vi "PinPointToRect.vi"(8 "错误输入":errorcluster, 10 "point":cluster{"x":i16, "y":i16} caption="点", 11 "rect":T2 caption="矩形") -> (0 "错误输出":errorcluster, 1 "edge":T1 caption="边缘", 2 "pinned point":cluster{"x":i16, "y":i16} caption="锁定点")   [LabVIEW 2012, in "Picture Box Tools.lvlib" / "Rect Tools.lvlib"]
uses:
  Rect Tools.lvlib
  EdgeEnum.ctl
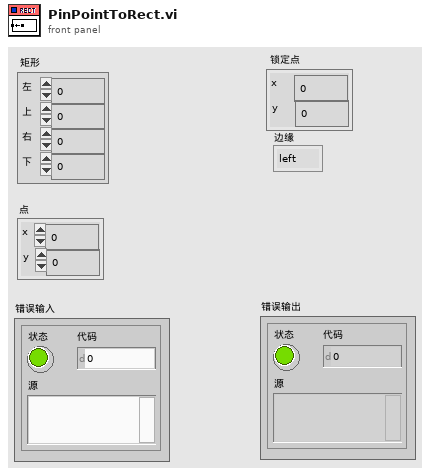
[diagram p1: front panel]
types:
  T1 = typedef "Picture Box Tools.lvlib/Rect Tools.lvlib/EdgeEnum.ctl" = enum16{"left", "top", "right", "bottom"}
  T2 = cluster{"left":i16, "top":i16, "right":i16, "bottom":i16}
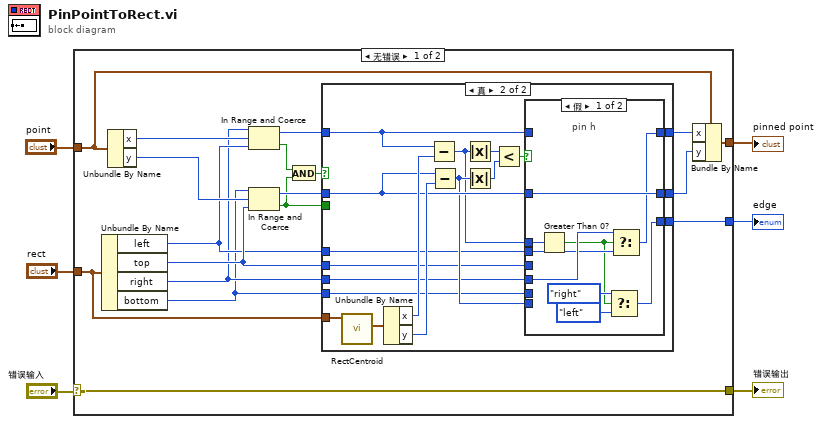
[diagram p0: block diagram]
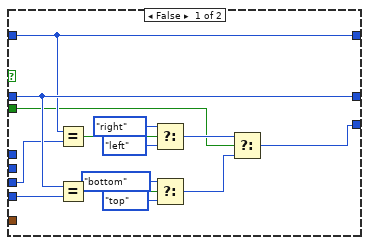
[diagram p2: hidden frame]
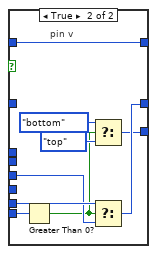
[diagram p3: hidden frame]
diagram:
  n1 = case shown="无错误" "错误输入" {
    selector: "错误输入" -> [w11 w75]
    tunnel: [w11 w75] -> w5
    tunnel: "point" -> [w10 _]
    tunnel: "rect" -> [w9 _]
    tunnel: [w8 _] -> w2
    tunnel: [w7 _] -> w1
    frame No Error {
      n2 = Unbundle By Name(w9) -> ("left"=w15:i16, "top"=w16:i16, "right"=w13:i16, "bottom"=w12:i16)
      n3 = Unbundle By Name(w10) -> ("x"=w24:i16, "y"=w23:i16)
      n4 = In Range and Coerce(upper limit=w13, x=w24, lower limit=w15) -> (coerced(x)=w20:i16, In Range?=w22:bool)
      n5 = In Range and Coerce(upper limit=w12, x=w23, lower limit=w16) -> (coerced(x)=w19:i16, In Range?=w14:bool)
      n6 = And(x=w22, y=w14) -> (x .and. y?=w21:bool)
      n7 = case shown="真" w21 {
        tunnel: w20 -> [w29 w48]
        tunnel: w19 -> [w34 w49]
        tunnel: [w29 w47] -> w18
        tunnel: [w34 w46] -> w17
        tunnel: w9 -> [_ w56]
        tunnel: w12 -> [w35 w40]
        tunnel: w16 -> [_ w42]
        tunnel: w13 -> [w30 w41]
        tunnel: w15 -> [_ w43]
        tunnel: [w26 w39] -> w7
        tunnel: w14 -> [w25 _]
        frame False {
          n8 = Equal?(x=w29, y=w30) -> (x = y?=w33:bool)
          n9 = Equal?(x=w34, y=w35) -> (x = y?=w36:bool)
          n10 = Select(t=EdgeEnum."right" ("edge"), s=w33, f=EdgeEnum."left" ("edge")) -> (s? t:f=w28:T1)
          n11 = Select(t=EdgeEnum."bottom" ("edge"), s=w36, f=EdgeEnum."top" ("edge")) -> (s? t:f=w27:T1)
          n12 = Select(t=w28, s=w25, f=w27) -> (s? t:f=w26:T1)
        }
        frame True {
          n13 = call "RectCentroid.vi"("Rect In"=w56) -> ("point"=w55:cluster{"x":i16, "y":i16})  [unwired: 8 in, 2 out]
          n14 = Unbundle By Name(w55) -> ("x"=w54:i16, "y"=w53:i16)
          n15 = Subtract(x=w48, y=w54) -> (x-y=w44:i16)
          n16 = Subtract(x=w49, y=w53) -> (x-y=w45:i16)
          n17 = Absolute Value(x=w44) -> (abs(x)=w51:i16)
          n18 = Absolute Value(x=w45) -> (abs(x)=w52:i16)
          n19 = Less?(x=w51, y=w52) -> (x < y?=w50:bool)
          n20 = case shown="假" w50 {
            tunnel: w49 -> [w65 _]
            tunnel: w48 -> [_ w74]
            tunnel: [w64 w74] -> w47
            tunnel: [w65 w73] -> w46
            tunnel: w45 -> [_ w72]
            tunnel: w40 -> [_ w71]
            tunnel: w42 -> [_ w70]
            tunnel: w44 -> [w63 _]
            tunnel: w41 -> [w62 _]
            tunnel: w43 -> [w61 _]
            tunnel: [w57 w66] -> w39
            frame False {
              # "pin h"
              n21 = Greater Than 0?(x=w63) -> (x > 0?=w58:bool)
              n22 = Select(t=EdgeEnum."right" ("edge"), s=w58, f=EdgeEnum."left" ("edge")) -> (s? t:f=w57:T1)
              n23 = Select(t=w62, s=w58, f=w61) -> (s? t:f=w64:i16)
            }
            frame True {
              # "pin v"
              n24 = Greater Than 0?(x=w72) -> (x > 0?=w67:bool)
              n25 = Select(t=EdgeEnum."bottom" ("edge"), s=w67, f=EdgeEnum."top" ("edge")) -> (s? t:f=w66:T1)
              n26 = Select(t=w71, s=w67, f=w70) -> (s? t:f=w73:i16)
            }
          }
        }
      }
      n27 = Bundle By Name(cluster=w10, "x"=w18, "y"=w17) -> (w8:cluster{"x":i16, "y":i16})
    }
    frame Error {
    }
  }
  "错误输出" <- w5
  "pinned point" <- w2
  "edge" <- w1
